vi "UnexpectedDepsCheck.vi"(6 "GUI Mode? {F)":bool, 7 "Failures Ref":refnum<vi>, 8 "error in (no error)":errorcluster, 9 "Status Indicator Ref":refnum<vi>, 10 "CheckChangedLibrariesOnly":bool=TRUE, 11 "Workspace Path":path=path "C:/sw-deps-monitor") -> (0 "error out":errorcluster, 2 "Status Indicator":string, 3 "Failures":T1[](array[typedef]))   [LabVIEW 2019, in "Hawkeye.lvlib"]
uses:
  Hawkeye.lvlib
  Typedefs/DepsCheckResult.ctl
  28450a76-a9d3-48c7-9439-369bd691228e.vi
  <vilib>/JDP Science/JSONtext/Variant to JSON Text.vi
  <vilib>/Wiresmith Technology/G CLI/CLI Class/CLI.lvclass
  <vilib>/JDP Science/JSONtext/LVClass Serializer/JSONtext LVClass Serializer.lvclass
  <vilib>/SLL Toolkit/SLL String/SLL String.lvlib
  <vilib>/JDP Science/JSONtext/JSONtext.lvlib
panel:
  in  "Tab Control":enum32{"GUI Mode", "CLI Mode"}(tab)
  out "Args":string[](array[string])=["C:\\sw-deps-monitor", "True"]
  # "When in GUI Mode, the controls will be used, \nIn CLI Mode, the Args will be used"
  # "Workspace Path"
  # "CheckChangedLibrariesOnly? True/False"
  # "Command to run the VI from terminal\ng-cli -v --lv-ver 2023 --arch 32 \"C:\\sw-deps-monitor\\CICD\\AutomatedChecks\\UnexpectedDepsCheck.vi\" -- \"C:\\sw-deps-monitor\" \"False\""
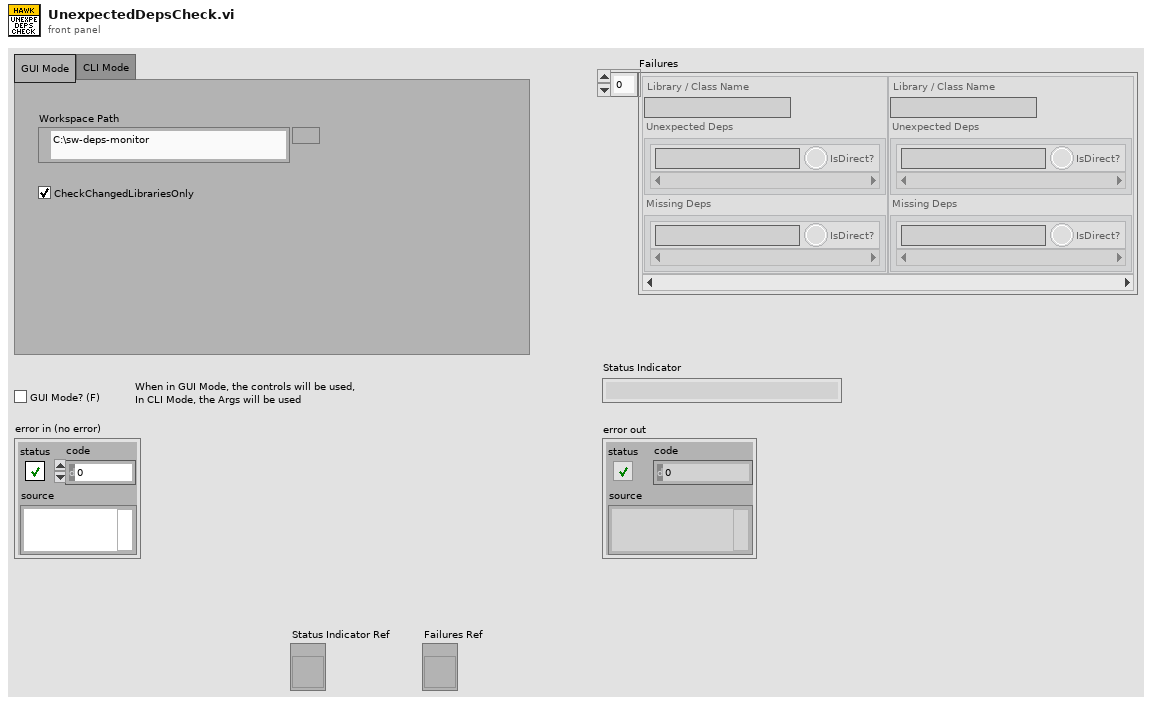
[diagram p1: front panel]
types:
  T1 = typedef "Hawkeye.lvlib/DepsCheckResult.ctl" = cluster{"Library / Class Name":string, "Unexpected Deps":cluster{"Dependency":string, "IsDirect?":bool}[], "Missing Deps":cluster{"Dependency":string, "IsDirect?":bool}[]}
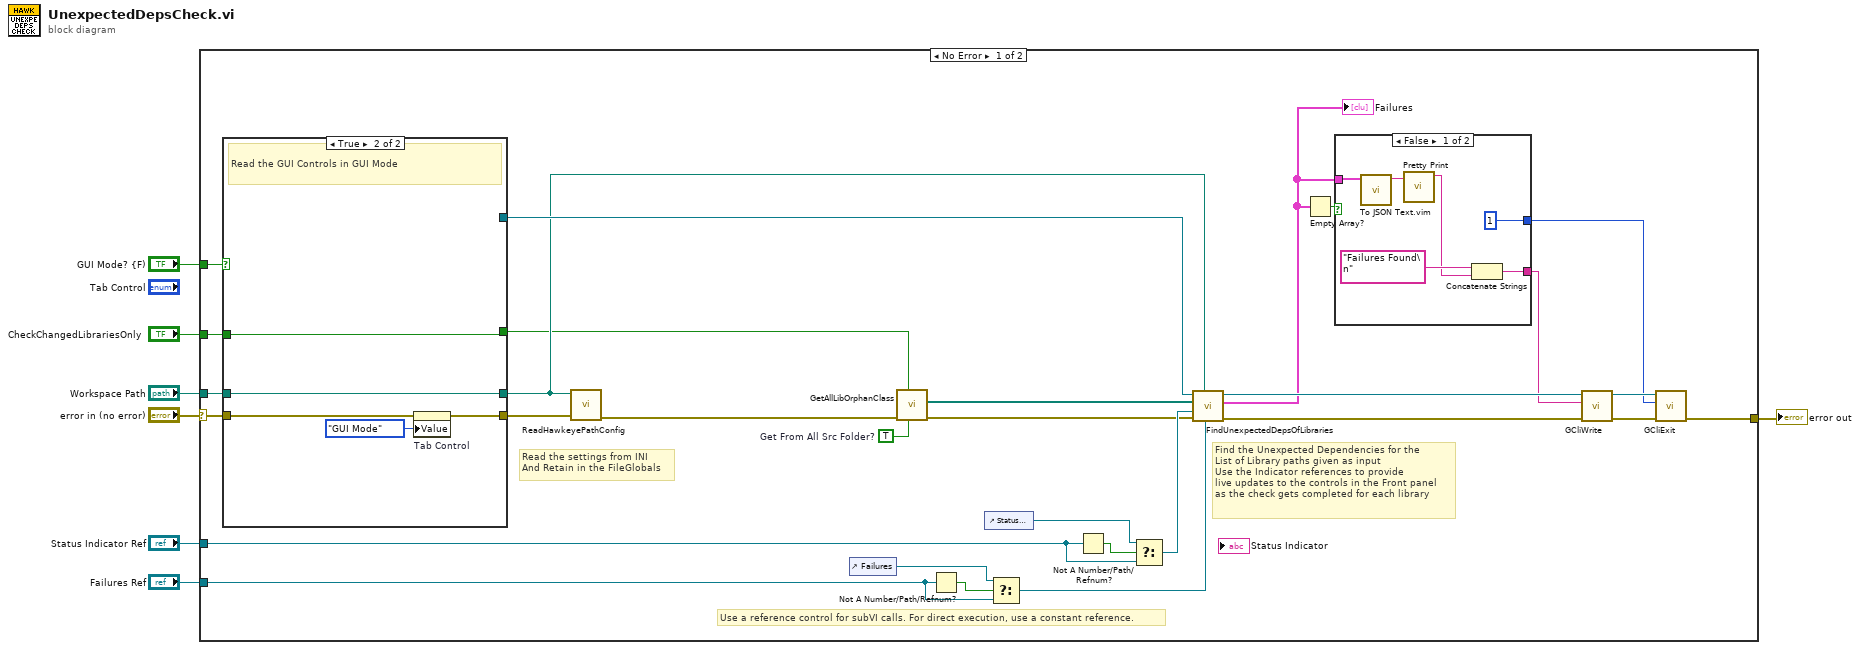
[diagram p0: block diagram]
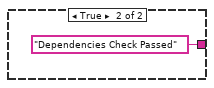
[diagram p2: hidden frame]
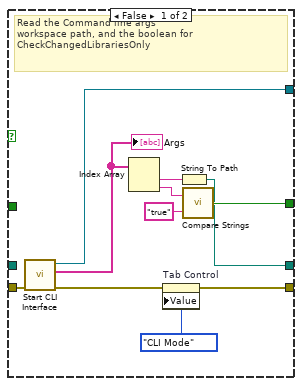
[diagram p3: hidden frame]
diagram:
  n1 = case shown="No Error" "error in (no error)" {
    selector: "error in (no error)" -> [w35 w60]
    tunnel: "GUI Mode? {F)" -> [w36 _]
    tunnel: [w26 w60] -> w5
    tunnel: "CheckChangedLibrariesOnly" -> [w24 _]
    tunnel: "Workspace Path" -> [w23 _]
    tunnel: "Status Indicator Ref" -> [w18 _]
    tunnel: "Failures Ref" -> [w14 _]
    frame No Error {
      w10 = TRUE  # Get From All Src Folder?
      # "Use a reference control for subVI calls. For direct execution, use a constant reference."
      # "Find the Unexpected Dependencies for the\nList of Library paths given as input\nUse the Indicator references to provide \nlive updates to the controls in the Front panel\nas the check gets completed for each library"
      # "Read the settings from INI\nAnd Retain in the FileGlobals"
      n2 = case shown="True" w36 {
        tunnel: w35 -> [w54 w59]
        tunnel: [w51 w58] -> w34
        tunnel: [w47 w56] -> w11
        tunnel: [w46 w55] -> w13
        tunnel: [w44 _] -> w33
        tunnel: w24 -> [_ w56]
        tunnel: w23 -> [_ w55]
        frame False {
          # "Read the Command line args\nworkspace path, and the boolean for\nCheckChangedLibrariesOnly"
          n3 = call <vilib>:"Start CLI Interface.vi"("error in (no error)"=w54) -> ("error out"=w53:errorcluster, "Custom Parameters"=w45:string[], "CLI out"=w44:refnum<class "CLI.lvclass">)  [unwired: 7 in, 1 out]
          "Args" <- w45
          n4 = Index Array(array=w45) -> (element #1=w50:string, element #2=w49:string)  [unwired: 2 in]
          n5 = property on="Tab Control" class="TabCtl (strict)"(error in=w53, "Value"=enum32{"GUI Mode", "CLI Mode"}."CLI Mode" ("Tab Control")) -> (error out=w51:errorcluster)  [unwired: 1 in, 1 out]
          n6 = String To Path(string=w50) -> (path=w46:path)
          n7 = call <vilib>:"Compare Strings.vi"("y"="true", "x"=w49) -> ("Equal?"=w47:bool)
        }
        frame True {
          # "Read the GUI Controls in GUI Mode"
          n8 = property on="Tab Control" class="TabCtl (strict)"(error in=w59, "Value"=enum32{"GUI Mode", "CLI Mode"}."GUI Mode" ("Tab Control")) -> (error out=w58:errorcluster)  [unwired: 1 in, 1 out]
        }
      }
      n9 = call "ReadHawkeyePathConfig.vi"("error in (no error)"=w34, "Workspace Path"=w13) -> ("error out"=w12:errorcluster)  [unwired: 8 in, 1 out]
      n10 = control-ref of="Failures"() -> (w16:refnum<vi>)
      n11 = call "GetAllLibOrphanClass.vi"("Get From All Src Folder?"=w10, "ListForChangedLibrariesOnly"=w11, "error in (no error)"=w12) -> ("error out"=w9:errorcluster, "Lib / Class Path []"=w8:path[])  [unwired: 6 in, 1 out]
      n12 = Not A Number/Path/Refnum?(number/path/refnum=w14) -> (NaN/Path/Refnum?=w17:bool)
      n13 = control-ref of="Status Indicator"() -> (w20:refnum<vi>)
      n14 = Select(t=w16, s=w17, f=w14) -> (s? t:f=w15:refnum<vi>)
      n15 = Not A Number/Path/Refnum?(number/path/refnum=w18) -> (NaN/Path/Refnum?=w21:bool)
      n16 = Select(t=w20, s=w21, f=w18) -> (s? t:f=w19:refnum<vi>)
      n17 = call "FindUnexpectedDepsOfLibraries.vi"("Failures Indicator Ref"=w15, "Workspace Path"=w13, "error in (no error)"=w9, "Status Indicator Ref"=w19, "Lvlib/Lvclass paths"=w8, "CLI in"=w33) -> ("error out"=w32:errorcluster, "Failures Array"=w22:T1[], "CLI out"=w30:refnum<class "CLI.lvclass">)  [unwired: 3 in]
      "Failures" <- w22
      n18 = Empty Array?(array=w22) -> (empty?=w28:bool)
      n19 = case shown="False" w28 {
        tunnel: w22 -> [w41 _]
        tunnel: [w40 "Dependencies Check Passed"] -> w27
        tunnel: [1 _] -> w25
        frame False {
          n20 = call "To JSON Text.vim"("Anything"=w41) -> ("<JSON>"=w38:string)  [unwired: 9 in, 1 out]
          n21 = call <vilib>:"Pretty Print.vi"("JSON"=w38) -> ("<JSON>"=w37:string)  [unwired: 8 in, 2 out]
          n22 = Concatenate Strings("Failures Found\n" ("string"), w37) -> (w40:string)
        }
        frame True {
        }
      }
      n23 = call "GCliWrite.vi"("error in (no error)"=w32, "Text to Write"=w27, "CLI in"=w30) -> ("error out"=w31:errorcluster, "CLI out"=w29:refnum<class "CLI.lvclass">)  [unwired: 7 in]
      n24 = call "GCliExit.vi"("error in (no error)"=w31, "No Error Code (0)"=w25, "CLI in"=w29) -> ("error out"=w26:errorcluster)  [unwired: 8 in]
    }
    frame Error {
    }
  }
  "error out" <- w5
